vi "TSM SSC Digital Apply TDR Offsets.vi"(0 "Digital TSM In":T1, 5 "Per-Instrument offsets (s)":dbl[][](array[numeric]), 11 "error in":errorcluster) -> (4 "Digital TSM Out":T1, 15 "error out":errorcluster)   [LabVIEW 2019]
doc: "Applies the correction for propagation delay offsets to digital pattern instrument(s) connected to the specified pin(s) and pin group(s).\n\nUse this VI to apply TDR offsets that are stored from a past measurement or are measured by means other than the niDigital TDR VI. Also use this VI to apply correction for offsets if the apply offsets input of the niDigital TDR VI was set to False at the time of measurement."
uses:
  TSM/TSM SSC Digital.ctl
  <vilib>/NI_TestStand_SemiconductorModule/NI_TestStand_Semiconductor_Module.lvlibp/PinMap/Digital Pattern/PinQueryContext/DigitalPatternPinQueryContext.lvclass
  SSC Digital/SSC Digital.ctl
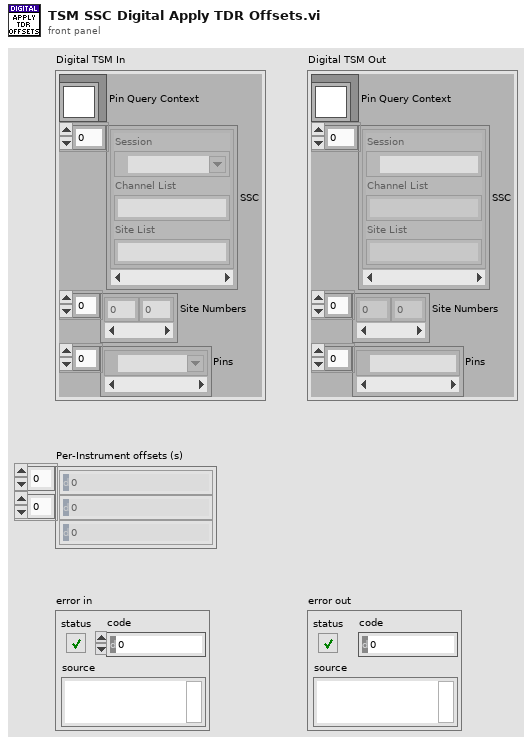
[diagram p1: front panel]
types:
  T1 = typedef "TSM SSC Digital.ctl" = cluster{"Pin Query Context":refnum<class "DigitalPatternPinQueryContext.lvclass">, "SSC":T2[], "Site Numbers":i32[], "Pins":tag[]}
  T2 = typedef "SSC Digital.ctl" = cluster{"Session":refnum<k15>, "Channel List":string, "Site List":string}
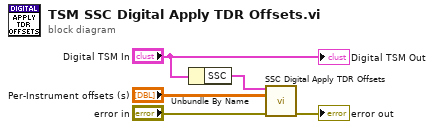
[diagram p0: block diagram]
diagram:
  n1 = Unbundle By Name("Digital TSM In") -> ("SSC"=w4:T2[])
  n2 = call "SSC Digital Apply TDR Offsets.vi"("Digital SSC in"=w4, "Per-Instrument offsets (s)"="Per-Instrument offsets (s)", "error in"="error in") -> ("error out"=→"error out":errorcluster)  [unwired: 11 in, 1 out]
  "Digital TSM Out" <- "Digital TSM In"
